vi "Check sensor str.vi"(7 "error in (no error)":errorcluster, 9 "Sensor value in":dbl, 10 "string":string) -> (0 "error out":errorcluster, 2 "Sensor value out":dbl)   [LabVIEW 2025, in "Control de MaP.lvlib"]
uses:
  Control de MaP.lvlib
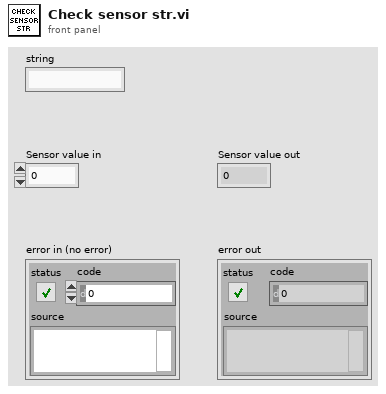
[diagram p1: front panel]
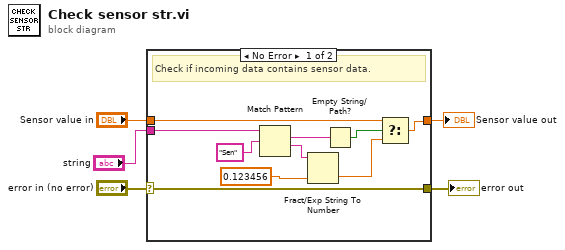
[diagram p0: block diagram]
diagram:
  n1 = case shown="No Error" "error in (no error)" {
    selector: "error in (no error)" -> [w8 w16]
    tunnel: [w15 w17] -> w5
    tunnel: "Sensor value in" -> [w12 w17]
    tunnel: [w8 w16] -> w2
    tunnel: "string" -> [w7 _]
    frame No Error {
      # "Check if incoming data contains sensor data."
      n2 = Match Pattern(string=w7, regular expression="Sen") -> (match substring=w10:string, after substring=w13:string)  [unwired: 1 in, 2 out]
      n3 = Fract/Exp String To Number(string=w13, default (0 dbl)=0.123456 ("default (0 DBL)")) -> (number=w14:dbl)  [unwired: 2 in, 1 out]
      n4 = Empty String/Path?(string/path=w10) -> (empty?=w11:bool)
      n5 = Select(t=w12, s=w11, f=w14) -> (s? t:f=w15:dbl)
    }
    frame Error {
    }
  }
  "Sensor value out" <- w5
  "error out" <- w2
